vi "Where.vi"(8 "error in (no error)":errorcluster, 11 "SQLite_API in":refnum<class "SQLite_API.lvclass">) -> (0 "error out":errorcluster, 3 "SQLite_API out":refnum<class "SQLite_API.lvclass">)   [LabVIEW 2021]
uses:
  <userlib>/John_Lib/DataBase/SQLite_API/SQLite_API.lvclass
  <userlib>/John_Lib/DataBase/SQLite_API/SQLite_API.lvclass/SQLite_API.ctl
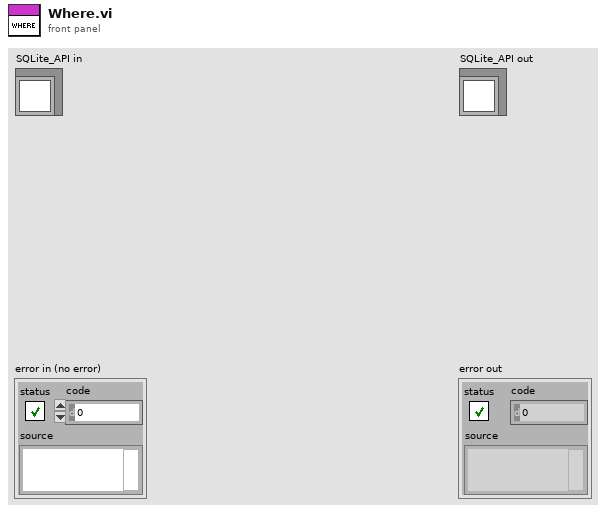
[diagram p1: front panel]
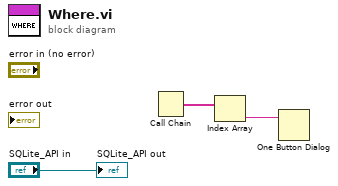
[diagram p0: block diagram]
diagram:
  n1 = Call Chain() -> (call chain=w1:string[])
  n2 = Index Array(array=w1) -> (element=w2:string)  [unwired: 1 in]
  n3 = One Button Dialog(message=w2) -> ()  [unwired: 1 in, 1 out]
  "SQLite_API out" <- "SQLite_API in"
